vi "gxml_BlindExtractData.vi"(8 "error in":errorcluster, 11 "XML Line":string) -> (0 "error out":errorcluster, 3 "Item Contents":string)   [LabVIEW 2009]
uses:
  <vilib>/regexp/Match Regular Expression.xnode
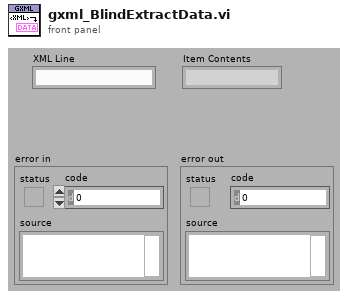
[diagram p1: front panel]
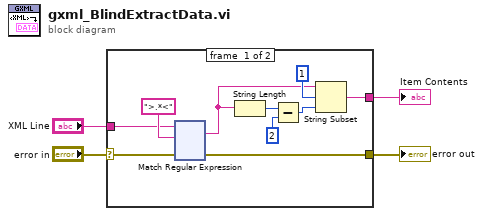
[diagram p0: block diagram]
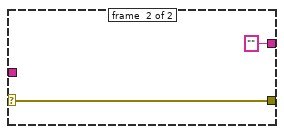
[diagram p2: hidden frame]
diagram:
  n1 = case shown="No Error" "error in" {
    selector: "error in" -> [w5 w123]
    tunnel: [w13 "" ("whole match")] -> w4
    tunnel: "XML Line" -> [w7 _]
    tunnel: [w6 w123] -> w2
    frame #0 {
      n2 = xnode "Match Regular Expression"("input string"=w7, "regular expression"=">.*<", "error in"=w5) -> ("whole match"=w9:string, "error out"=w6:errorcluster)  [unwired: 3 in, 3 out]
      n3 = String Length(string=w9) -> (length=w10:i32)
      n4 = Subtract(x=w10, y=2) -> (x-y=w12:i32)
      n5 = String Subset(string=w9, offset (0)=1, length (rest)=w12) -> (substring=w13:string)
    }
    frame #1 {
    }
  }
  "Item Contents" <- w4
  "error out" <- w2
